vi "Read Thermometer.vi"() -> ()   [LabVIEW 2020]
panel:
  out "Waveform Chart":dbl(graph)
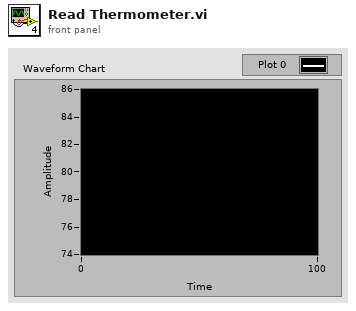
[diagram p1: front panel]
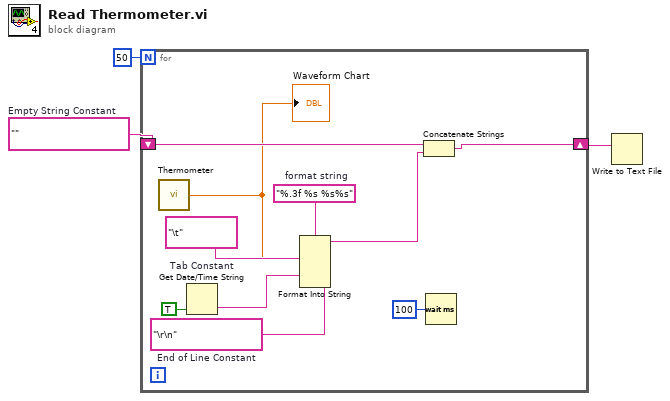
[diagram p0: block diagram]
diagram:
  w2 = ""  # Empty String Constant
  n1 = for {
    N: 50 -> [_]
    shift-right: [w7] -> w1
    shift-left: w2 -> [w9]
    w10 = "\r\n"  # End of Line Constant
    w6 = "\t"  # Tab Constant
    w13 = "%.3f %s %s%s"  # format string
    n2 = call "Thermometer.vi"() -> ("Temperature (deg F)"=w5:dbl)  [unwired: 1 in]
    "Waveform Chart" <- w5
    n3 = Get Date/Time String(want seconds? (F)=TRUE) -> (time string=w11:string)  [unwired: 2 in, 1 out]
    n4 = Format Into String "Format Into String"(format string=w13, w5, w6, w11, w10) -> (resulting string=w8:string)  [unwired: 2 in, 1 out]
    n5 = Concatenate Strings "Concatenate Strings"(w9, w8) -> (w7:string)
    n6 = Wait (ms)(milliseconds to wait=u32 100) -> ()  [unwired: 1 out]
  }
  n7 = Write to Text File(text=w1) -> ()  [unwired: 3 in, 3 out]
